vi "Gauge (Silver).vi"() -> ()   [LabVIEW 2012]
panel:
  out "Gauge":dbl(knob) scale=0.0..10.0
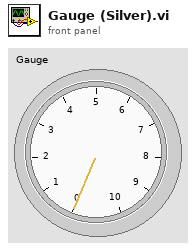
[diagram p1: front panel]
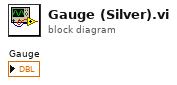
[diagram p0: block diagram]
diagram:
